vi "feature locator.vi"(1 "Features":dbl[](array[numeric]), 2 "Locations":dbl[](array[numeric])) -> (0 "Feature locations":dbl[](array[numeric]))   [LabVIEW 2014]
panel:
  # "Processes peak data to find the nearest matching \nlocation within the spectrum"
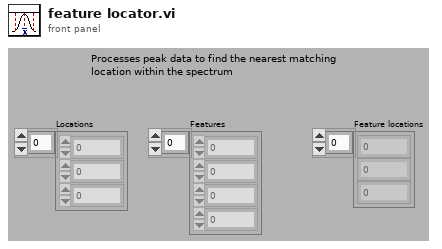
[diagram p1: front panel]
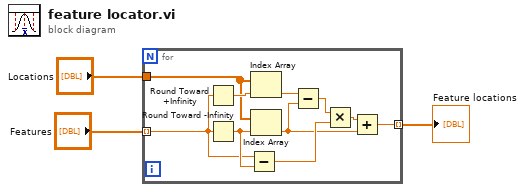
[diagram p0: block diagram]
diagram:
  n1 = for {
    tunnel: "Features" -> [w10] mode=indexing
    tunnel: "Locations" -> [w12]
    tunnel: [w4] -> w3 mode=indexing
    n2 = Round Toward +Infinity ("Round To +Infinity")(x=w10) -> (ceil(x): smallest int >= x=w13:dbl)
    n3 = Round Toward -Infinity ("Round To -Infinity")(1:w10) -> (0:w11:dbl)
    n4 = Subtract(x=w10, y=w11) -> (x-y=w7:dbl)
    n5 = Index Array(array=w12, index=w13) -> (element=w9:dbl)
    n6 = Index Array(array=w12, index=w11) -> (element=w5:dbl)
    n7 = Subtract(x=w9, y=w5) -> (x-y=w8:dbl)
    n8 = Multiply(x=w8, y=w7) -> (x*y=w6:dbl)
    n9 = Add(x=w6, y=w5) -> (x+y=w4:dbl)
  }
  "Feature locations" <- w3
